vi "6_Area and Circumference of a circle.vi"() -> ()   [LabVIEW 2018]
panel:
  out "Circumference":dbl
  out "AREA":dbl
  in  "RADIUS":dbl
  # "WAP to find area and circumference of a circle"
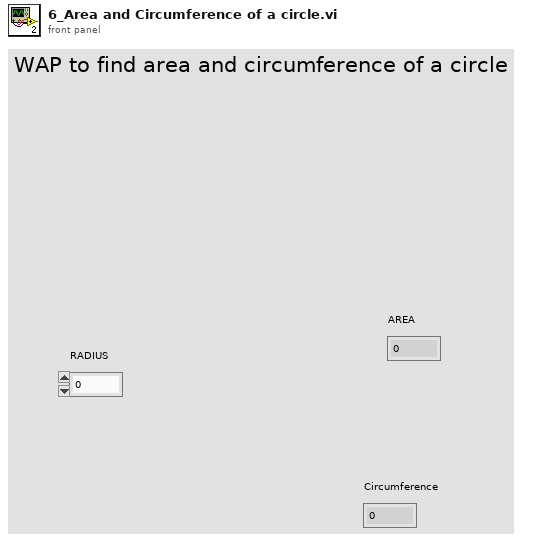
[diagram p1: front panel]
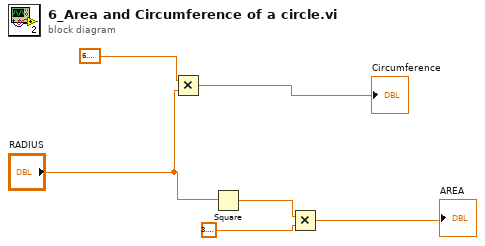
[diagram p0: block diagram]
diagram:
  n1 = Multiply(x=6.283185307179586, y="RADIUS") -> (x*y=→"Circumference":dbl)
  n2 = Square(x="RADIUS") -> (x^2=w6:dbl)
  n3 = Multiply(x=w6, y=3.141592653589793) -> (x*y=→"AREA":dbl)
